vi "StartAModule.vi"(7 "ShowPanel?":bool, 8 "Error Array In":errorcluster[](array[cluster]), 11 "Module Name (Sensor, Fgen, etc.)":string) -> (0 "ErrorArray Out":errorcluster[](array[cluster]), 1 "Variant":variant, 2 "Clone Registration":refnum<data-value>, 3 "Module ID":i32)   [LabVIEW 2018, in "Test.lvclass"]
uses:
  Test.lvclass
  <userlib>/NIST/ModuleAdminLib/CloneRegistration/CloneRegistration.lvclass
  <userlib>/NIST/ModuleAdminLib/ModuleAdmin/ModuleAdmin.lvclass/ModuleAdmin.ctl
  <userlib>/NIST/ModuleAdminLib/ModuleAdmin/Accessors/Read CloneRegRef.vi
  Sync/SyncModule/Main.vi
  FGen/FgenPlugins/Main.vi
  Analysis/AnalysisModule/Main.vi
  AcPwr/AcPwrPlugins/Common/Main.vi
  <vilib>/Utility/error.llb/Error Cluster From Error Code.vi
  <vilib>/ErrorRing/Error Ring.xnode
  <userlib>/NIST/ModuleAdminLib/ModuleAdmin/ModuleAdmin.lvclass
  Sync/SyncModule/SyncModule.lvlib
  <userlib>/NIST/NISTErrorLib/NISTErrorLib.lvlib
  FGen/FgenPlugins/FgenPlugins.lvlib
  FGen/FgenShared/FgenShared.lvlib
  Digitizer/DigitizerShared/DigitizerShared.lvlib
  Scope/ScopeShared/ScopeShared.lvlib
  Sensor/SensorShared/SensorShared.lvlib
  Analysis/AnalysisModule/AnalysisModule.lvlib
  AcPwr/AcPwrShared/AcPwrShared.lvlib
  AcPwr/AcPwrPlugins/AcPwrPlugins.lvlib
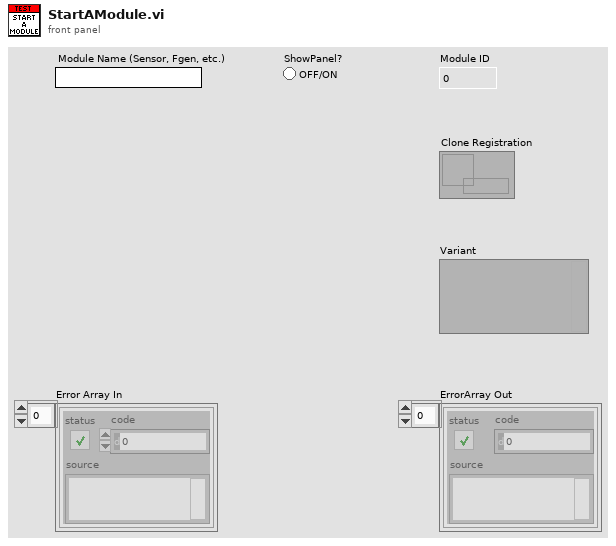
[diagram p1: front panel]
types:
  T1 = typedef "SyncModule.lvlib/SyncBroadcastEvents.ctl" = cluster{"DidInit":refnum<user-event>, "StatusUpdate":refnum<user-event>, "ErrorReport":refnum<user-event>, "DidStop":refnum<user-event>, "PathToINI":refnum<user-event>, "TriggerTime":refnum<user-event>, "LockStatus":refnum<user-event>, "Info":refnum<user-event>, "ClockProperties":refnum<user-event>, "SyncData":refnum<user-event>, "TimingSession":refnum<user-event>}
  T2 = typedef "FgenShared.lvlib/clBroadcastEvents.ctl" = cluster{"DidInit":refnum<user-event>, "StatusUpdate":refnum<user-event>, "ErrorReport":refnum<user-event>, "DidStop":refnum<user-event>, "PathToINI":refnum<user-event>, "Channels":refnum<user-event>, "Function":refnum<user-event>, "Waveforms":refnum<user-event>, "Triggers":refnum<user-event>, "FunctionParams":refnum<user-event>, "FunctionArbs":refnum<user-event>, "FunctionSampleRate":refnum<user-event>}
  T3 = typedef "DigitizerShared.lvlib/clBroadcastEvents.ctl" = cluster{"DidInit":refnum<user-event>, "StatusUpdate":refnum<user-event>, "ErrorReport":refnum<user-event>, "DidStop":refnum<user-event>, "PathToINI":refnum<user-event>, "Channels":refnum<user-event>, "Acq":refnum<user-event>, "Trigger":refnum<user-event>, "Waveforms":refnum<user-event>}
  T4 = typedef "ScopeShared.lvlib/clBroadcastEvents.ctl" = cluster{"DidInit":refnum<user-event>, "StatusUpdate":refnum<user-event>, "ErrorReport":refnum<user-event>, "DidStop":refnum<user-event>, "PathToINI":refnum<user-event>, "Handle":refnum<user-event>, "Model":refnum<user-event>, "Channels":refnum<user-event>, "Acquisition":refnum<user-event>, "Trigger":refnum<user-event>, "ExtAcquisition":refnum<user-event>, "Waveform":refnum<user-event>}
  T5 = typedef "SensorShared.lvlib/clBroadcastEvents.ctl" = cluster{"DidInit":refnum<user-event>, "StatusUpdate":refnum<user-event>, "ErrorReport":refnum<user-event>, "DidStop":refnum<user-event>, "PathToINI":refnum<user-event>, "SensorReport":refnum<user-event>, "SensorConfig":refnum<user-event>}
  T6 = typedef "AnalysisModule.lvlib/clBroadcastEvents.ctl" = cluster{"DidInit":refnum<user-event>, "StatusUpdate":refnum<user-event>, "ErrorReport":refnum<user-event>, "DidStop":refnum<user-event>, "PathToINI":refnum<user-event>, "Config":refnum<user-event>, "ResultReport":refnum<user-event>, "FunctionClass":refnum<user-event>, "State":refnum<user-event>, "FunctionParams":refnum<user-event>, "Duration":refnum<user-event>}
  T7 = typedef "AcPwrShared.lvlib/AcPwrBroadcastEvents.ctl" = cluster{"DidInit":refnum<user-event>, "StatusUpdate":refnum<user-event>, "ErrorReport":refnum<user-event>, "DidStop":refnum<user-event>, "PathToINI":refnum<user-event>, "Measurements":refnum<user-event>, "LoadConfigFile":refnum<user-event>, "GetSettings":refnum<user-event>, "SetSettings":refnum<user-event>, "GetType&ID":refnum<user-event>, "GotSettings":refnum<user-event>, "GotSettingsLV":refnum<user-event>}
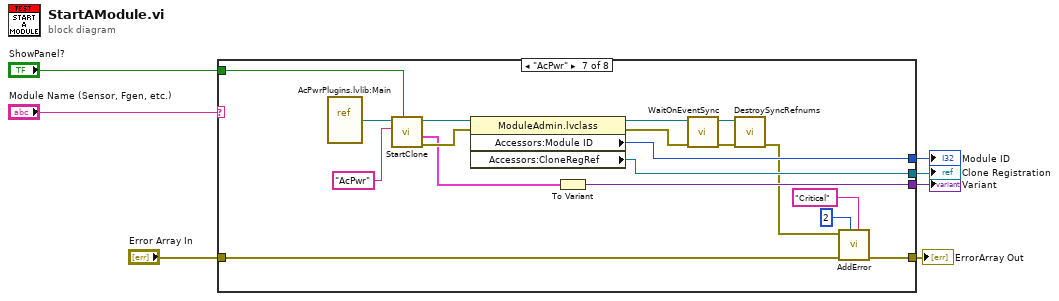
[diagram p0: block diagram]
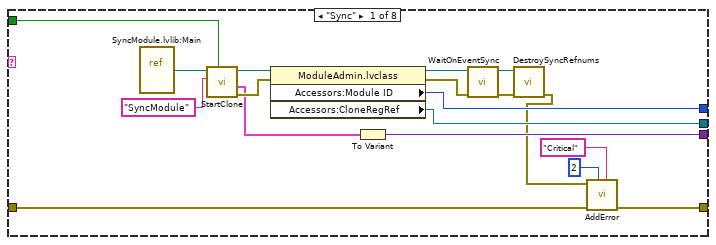
[diagram p2: hidden frame]
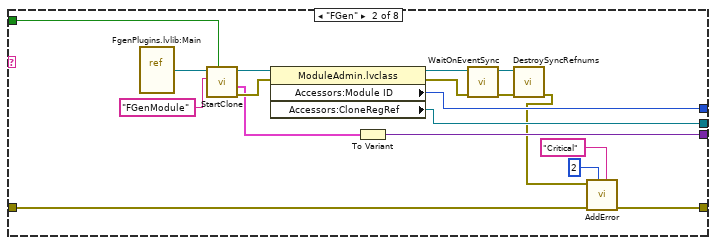
[diagram p3: hidden frame]
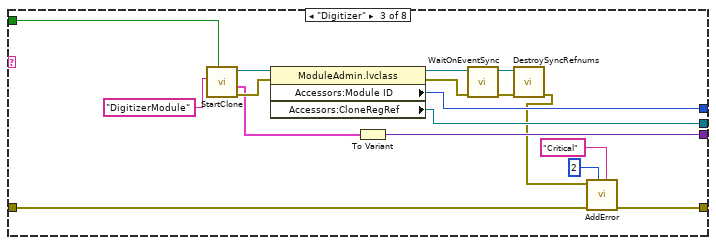
[diagram p4: hidden frame]
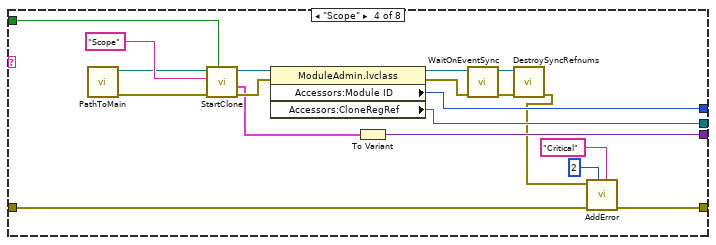
[diagram p5: hidden frame]
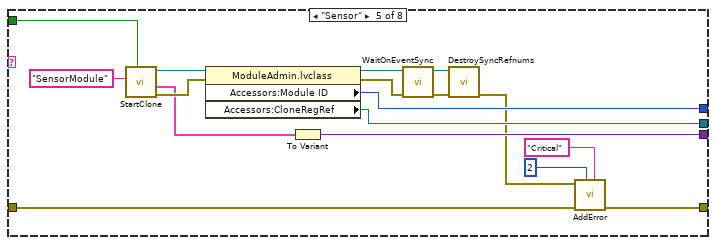
[diagram p6: hidden frame]
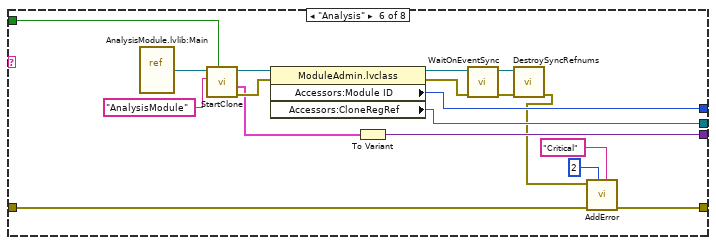
[diagram p7: hidden frame]
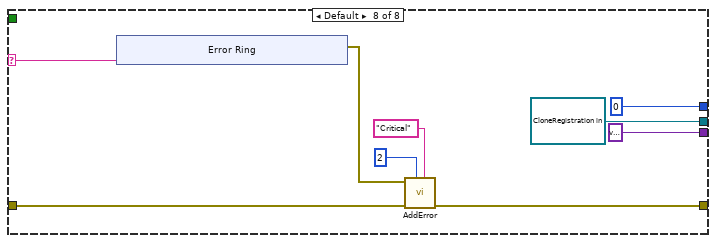
[diagram p8: hidden frame]
diagram:
  n1 = case shown="\"AcPwr\"" "Module Name (Sensor, Fgen, etc.)" {
    selector: "Module Name (Sensor, Fgen, etc.)" -> [_ _ _ _ _ _ _ w141]
    tunnel: "Error Array In" -> [w10 w28 w46 w65 w82 w99 w118 w140]
    tunnel: [w13 w31 w49 w68 w85 w102 w121 w136] -> w2
    tunnel: [w14 w32 w50 w69 w86 w103 w122 variant ("Variant")] -> w3
    tunnel: [w16 w34 w52 w71 w88 w105 w124 refnum<data-value> refnum ("Accessors:CloneRegRef")] -> w4
    tunnel: [w15 w33 w51 w70 w87 w104 w123 0 ("Accessors:Module ID")] -> w5
    tunnel: "ShowPanel?" -> [w8 w26 w44 w63 w80 w97 w116 _]
    frame "Sync" {
      n2 = vi-ref "SyncModule.lvlib:Main.vi"() -> (w25:refnum<vi>)
      n3 = call "StartClone.vi"("ShowPanel? (f)"=w8, "ModuleName"="SyncModule", "VI Refnum"=w25) -> ("error out"=w18:errorcluster, "SyncBroadcastEvents"=w17:T1, "ModuleAdmin"=w23:refnum<class "ModuleAdmin.lvclass">)  [unwired: 6 in]
      n4 = property class="ModuleAdmin.lvclass"(reference=w23, error in=w18) -> (reference out=w21:refnum<class "ModuleAdmin.lvclass">, error out=w22:errorcluster, "Accessors:Module ID"=w15:i32, "Accessors:CloneRegRef"=w16:refnum<data-value>)
      n5 = To Variant(anything=w17) -> (Variant=w14:variant)
      n6 = call <userlib>:"WaitOnEventSync.vi"("error in (no error)"=w22, "ModuleAdmin"=w21) -> ("error out"=w20:errorcluster, "ModuleAdmin"=w19:refnum<class "ModuleAdmin.lvclass">)  [unwired: 8 in]
      n7 = call <userlib>:"DestroySyncRefnums.vi"("error in (no error)"=w20, "ModuleAdmin"=w19) -> ("error out"=w9:errorcluster)  [unwired: 9 in]
      n8 = call <userlib>:"AddError.vi"("Severity"="Critical", "Priority"=u8 2, "ErrorArray In"=w10, "error in (no error)"=w9) -> ("ErrorArray Out"=w13:errorcluster[])  [unwired: 6 in, 1 out]
    }
    frame "FGen" {
      n9 = vi-ref "FgenPlugins.lvlib:Main.vi"() -> (w43:refnum<vi>)
      n10 = call "StartClone.vi"("ShowPanel? (f)"=w26, "ModuleName"="FGenModule", "VI Refnum"=w43) -> ("error out"=w36:errorcluster, "clBroadcastEvents"=w35:T2, "ModuleAdmin"=w41:refnum<class "ModuleAdmin.lvclass">)  [unwired: 6 in]
      n11 = property class="ModuleAdmin.lvclass"(reference=w41, error in=w36) -> (reference out=w39:refnum<class "ModuleAdmin.lvclass">, error out=w40:errorcluster, "Accessors:Module ID"=w33:i32, "Accessors:CloneRegRef"=w34:refnum<data-value>)
      n12 = To Variant(anything=w35) -> (Variant=w32:variant)
      n13 = call <userlib>:"WaitOnEventSync.vi"("error in (no error)"=w40, "ModuleAdmin"=w39) -> ("error out"=w38:errorcluster, "ModuleAdmin"=w37:refnum<class "ModuleAdmin.lvclass">)  [unwired: 8 in]
      n14 = call <userlib>:"DestroySyncRefnums.vi"("error in (no error)"=w38, "ModuleAdmin"=w37) -> ("error out"=w27:errorcluster)  [unwired: 9 in]
      n15 = call <userlib>:"AddError.vi"("Severity"="Critical", "Priority"=u8 2, "ErrorArray In"=w28, "error in (no error)"=w27) -> ("ErrorArray Out"=w31:errorcluster[])  [unwired: 6 in, 1 out]
    }
    frame "Digitizer" {
      n16 = call "StartClone.vi"("ShowPanel? (f)"=w44, "ModuleName"="DigitizerModule") -> ("error out"=w54:errorcluster, "clBroadcastEvents"=w53:T3, "ModuleAdmin"=w59:refnum<class "ModuleAdmin.lvclass">)  [unwired: 7 in]
      n17 = property class="ModuleAdmin.lvclass"(reference=w59, error in=w54) -> (reference out=w57:refnum<class "ModuleAdmin.lvclass">, error out=w58:errorcluster, "Accessors:Module ID"=w51:i32, "Accessors:CloneRegRef"=w52:refnum<data-value>)
      n18 = To Variant(anything=w53) -> (Variant=w50:variant)
      n19 = call <userlib>:"WaitOnEventSync.vi"("error in (no error)"=w58, "ModuleAdmin"=w57) -> ("error out"=w56:errorcluster, "ModuleAdmin"=w55:refnum<class "ModuleAdmin.lvclass">)  [unwired: 8 in]
      n20 = call <userlib>:"DestroySyncRefnums.vi"("error in (no error)"=w56, "ModuleAdmin"=w55) -> ("error out"=w45:errorcluster)  [unwired: 9 in]
      n21 = call <userlib>:"AddError.vi"("Severity"="Critical", "Priority"=u8 2, "ErrorArray In"=w46, "error in (no error)"=w45) -> ("ErrorArray Out"=w49:errorcluster[])  [unwired: 6 in, 1 out]
    }
    frame "Scope" {
      n22 = call "PathToMain.vi"() -> ("Error Out"=w62:errorcluster, "PathToMain"=w61:path)  [unwired: 10 in]
      n23 = call "StartClone.vi"("ShowPanel? (f)"=w63, "error in (no error)"=w62, "ModuleName"="Scope", "vi path"=w61) -> ("error out"=w73:errorcluster, "clBroadcastEvents"=w72:T4, "ModuleAdmin"=w78:refnum<class "ModuleAdmin.lvclass">)  [unwired: 5 in]
      n24 = property class="ModuleAdmin.lvclass"(reference=w78, error in=w73) -> (reference out=w76:refnum<class "ModuleAdmin.lvclass">, error out=w77:errorcluster, "Accessors:Module ID"=w70:i32, "Accessors:CloneRegRef"=w71:refnum<data-value>)
      n25 = To Variant(anything=w72) -> (Variant=w69:variant)
      n26 = call <userlib>:"WaitOnEventSync.vi"("error in (no error)"=w77, "ModuleAdmin"=w76) -> ("error out"=w75:errorcluster, "ModuleAdmin"=w74:refnum<class "ModuleAdmin.lvclass">)  [unwired: 8 in]
      n27 = call <userlib>:"DestroySyncRefnums.vi"("error in (no error)"=w75, "ModuleAdmin"=w74) -> ("error out"=w64:errorcluster)  [unwired: 9 in]
      n28 = call <userlib>:"AddError.vi"("Severity"="Critical", "Priority"=u8 2, "ErrorArray In"=w65, "error in (no error)"=w64) -> ("ErrorArray Out"=w68:errorcluster[])  [unwired: 6 in, 1 out]
    }
    frame "Sensor" {
      n29 = call "StartClone.vi"("ShowPanel? (f)"=w80, "ModuleName"="SensorModule") -> ("error out"=w90:errorcluster, "clBroadcastEvents"=w89:T5, "ModuleAdmin"=w95:refnum<class "ModuleAdmin.lvclass">)  [unwired: 7 in]
      n30 = property class="ModuleAdmin.lvclass"(reference=w95, error in=w90) -> (reference out=w93:refnum<class "ModuleAdmin.lvclass">, error out=w94:errorcluster, "Accessors:Module ID"=w87:i32, "Accessors:CloneRegRef"=w88:refnum<data-value>)
      n31 = To Variant(anything=w89) -> (Variant=w86:variant)
      n32 = call <userlib>:"WaitOnEventSync.vi"("error in (no error)"=w94, "ModuleAdmin"=w93) -> ("error out"=w92:errorcluster, "ModuleAdmin"=w91:refnum<class "ModuleAdmin.lvclass">)  [unwired: 8 in]
      n33 = call <userlib>:"DestroySyncRefnums.vi"("error in (no error)"=w92, "ModuleAdmin"=w91) -> ("error out"=w81:errorcluster)  [unwired: 9 in]
      n34 = call <userlib>:"AddError.vi"("Severity"="Critical", "Priority"=u8 2, "ErrorArray In"=w82, "error in (no error)"=w81) -> ("ErrorArray Out"=w85:errorcluster[])  [unwired: 6 in, 1 out]
    }
    frame "Analysis" {
      n35 = vi-ref "AnalysisModule.lvlib:Main.vi"() -> (w114:refnum<vi>)
      n36 = call "StartClone.vi"("ShowPanel? (f)"=w97, "ModuleName"="AnalysisModule", "VI Refnum"=w114) -> ("error out"=w107:errorcluster, "AnalysisBroadcastEvents"=w106:T6, "ModuleAdmin"=w112:refnum<class "ModuleAdmin.lvclass">)  [unwired: 6 in]
      n37 = property class="ModuleAdmin.lvclass"(reference=w112, error in=w107) -> (reference out=w110:refnum<class "ModuleAdmin.lvclass">, error out=w111:errorcluster, "Accessors:Module ID"=w104:i32, "Accessors:CloneRegRef"=w105:refnum<data-value>)
      n38 = To Variant(anything=w106) -> (Variant=w103:variant)
      n39 = call <userlib>:"WaitOnEventSync.vi"("error in (no error)"=w111, "ModuleAdmin"=w110) -> ("error out"=w109:errorcluster, "ModuleAdmin"=w108:refnum<class "ModuleAdmin.lvclass">)  [unwired: 8 in]
      n40 = call <userlib>:"DestroySyncRefnums.vi"("error in (no error)"=w109, "ModuleAdmin"=w108) -> ("error out"=w98:errorcluster)  [unwired: 9 in]
      n41 = call <userlib>:"AddError.vi"("Severity"="Critical", "Priority"=u8 2, "ErrorArray In"=w99, "error in (no error)"=w98) -> ("ErrorArray Out"=w102:errorcluster[])  [unwired: 6 in, 1 out]
    }
    frame "AcPwr" {
      n42 = vi-ref "AcPwrPlugins.lvlib:Main.vi"() -> (w115:refnum<vi>)
      n43 = call "StartClone.vi"("ShowPanel? (f)"=w116, "ModuleName"="AcPwr", "VI Refnum"=w115) -> ("error out"=w126:errorcluster, "clAcPwrEvents"=w125:T7, "ModuleAdmin"=w131:refnum<class "ModuleAdmin.lvclass">)  [unwired: 6 in]
      n44 = property class="ModuleAdmin.lvclass"(reference=w131, error in=w126) -> (reference out=w129:refnum<class "ModuleAdmin.lvclass">, error out=w130:errorcluster, "Accessors:Module ID"=w123:i32, "Accessors:CloneRegRef"=w124:refnum<data-value>)
      n45 = To Variant(anything=w125) -> (Variant=w122:variant)
      n46 = call <userlib>:"WaitOnEventSync.vi"("error in (no error)"=w130, "ModuleAdmin"=w129) -> ("error out"=w128:errorcluster, "ModuleAdmin"=w127:refnum<class "ModuleAdmin.lvclass">)  [unwired: 8 in]
      n47 = call <userlib>:"DestroySyncRefnums.vi"("error in (no error)"=w128, "ModuleAdmin"=w127) -> ("error out"=w117:errorcluster)  [unwired: 9 in]
      n48 = call <userlib>:"AddError.vi"("Severity"="Critical", "Priority"=u8 2, "ErrorArray In"=w118, "error in (no error)"=w117) -> ("ErrorArray Out"=w121:errorcluster[])  [unwired: 6 in, 1 out]
    }
    frame Default {
      n49 = xnode "Error Ring"("parameter 0"=w141) -> ("error out"=w139:errorcluster)
      n50 = call <userlib>:"AddError.vi"("Severity"="Critical", "Priority"=u8 2, "ErrorArray In"=w140, "error in (no error)"=w139) -> ("ErrorArray Out"=w136:errorcluster[])  [unwired: 6 in, 1 out]
    }
  }
  "Module ID" <- w5
  "Clone Registration" <- w4
  "Variant" <- w3
  "ErrorArray Out" <- w2
